vi "Create Custom element (fixed_coords).vi"(7 "Type (Input)":T1, 8 "error in":errorcluster, 9 "type":string, 10 "name":string, 11 "Item Ref in":T2 format="%.0x") -> (0 "error out":errorcluster, 3 "Item Ref out":T2 format="%.0x")   [LabVIEW 2019, in "HLA Custom Device System Explorer.lvlib"]
uses:
  HLA Custom Device System Explorer.lvlib
  <vilib>/NI VeriStand/Custom Device API/Custom Device Item Ref.ctl
  <vilib>/NI VeriStand/Custom Device API/Custom Device Channel Type.ctl
  <vilib>/NI VeriStand/Custom Device API/Custom Device Channel.ctl
  Shared/Constants.vi
  <vilib>/NI VeriStand/Custom Device API/Custom Device API.lvlib
  Shared/HLA Custom Device Shared.lvlib
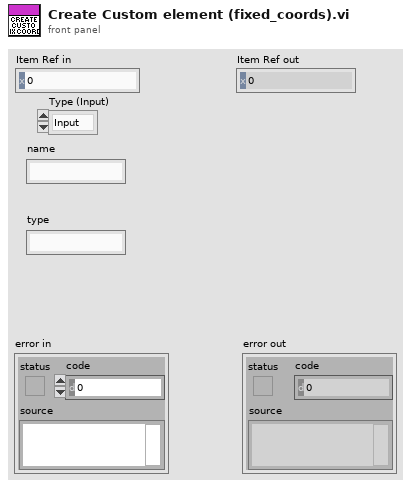
[diagram p1: front panel]
types:
  T1 = typedef "Custom Device API.lvlib/Custom Device Channel Type.ctl" = enum16{"Input", "Output"}
  T2 = typedef "Custom Device API.lvlib/Custom Device Item Ref.ctl" = u64
  T3 = typedef "Custom Device API.lvlib/Custom Device Channel.ctl" = cluster{"Type":T1, "Units":string, "Default Value":dbl, "Faultable":bool, "Scalable":bool}
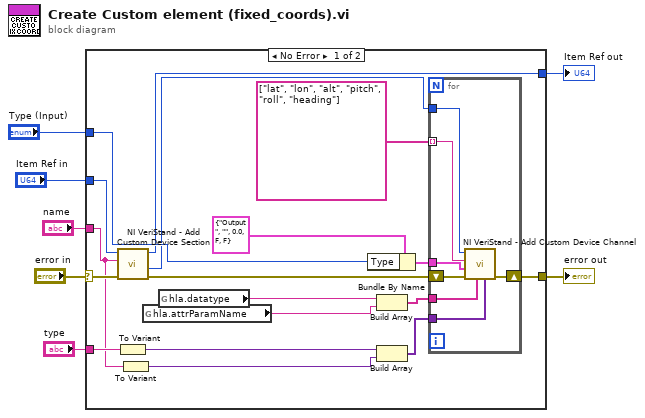
[diagram p0: block diagram]
diagram:
  n1 = case shown="No Error" "error in" {
    selector: "error in" -> [w16 w33]
    tunnel: [w20 w33] -> w6
    tunnel: [w14 w34] -> w5
    tunnel: "Item Ref in" -> [w15 w34]
    tunnel: "name" -> [w9 _]
    tunnel: "type" -> [w19 _]
    tunnel: "Type (Input)" -> [w17 _]
    frame No Error {
      n2 = call <vilib>:"NI VeriStand - Add Custom Device Section.vi"("error in (no error)"=w16, "Section Name"=w9, "Parent Ref in"=w15) -> ("error out"=w13:errorcluster, "Section Ptr"=w11:T2, "Parent Ref out"=w14:T2)  [unwired: 5 in, 1 out]
      n3 = To Variant(anything=w19) -> (Variant=w25:variant)
      n4 = To Variant(anything=w9) -> (Variant=w8:variant)
      n5 = global read "Constants.vi" "hla.attrParamName"() -> (w10:string)
      n6 = global read "Constants.vi" "hla.datatype"() -> (w23:string)
      n7 = Bundle By Name(cluster=T3 {"Type"=enum."Output", "Units"="", "Default Value"=0.0, "Faultable"=FALSE, "Scalable"=FALSE} ("Channel"), "Type"=w17) -> (w18:T3)
      n8 = Build Array(w23, w10) -> (w22:string[])
      n9 = Build Array(w25, w8) -> (w24:variant[])
      n10 = for {
        tunnel: w24 -> [w32]
        tunnel: w22 -> [w31]
        tunnel: w18 -> [w29]
        shift-right: [w30] -> w20
        shift-left: w13 -> [w28]
        tunnel: string[] ["lat", "lon", "alt", "pitch", "roll", "heading"] -> [w27] mode=indexing
        tunnel: w11 -> [w26]
        n11 = call <vilib>:"NI VeriStand - Add Custom Device Channel.vi"("Property Values"=w32, "Property names"=w31, "error in (no error)"=w28, "Channel"=w29, "Channel Name"=w27, "Parent Ref in"=w26) -> ("error out"=w30:errorcluster)  [unwired: 2 in, 3 out]
      }
    }
    frame Error {
    }
  }
  "error out" <- w6
  "Item Ref out" <- w5
